vi "circ_ap && file_pgm.vi"() -> ()   [LabVIEW 2012, in "LightPipes.lvlib"]
uses:
  LightPipes.lvlib
panel:
  in  "n_grid":i32=256
  out "field out":T1
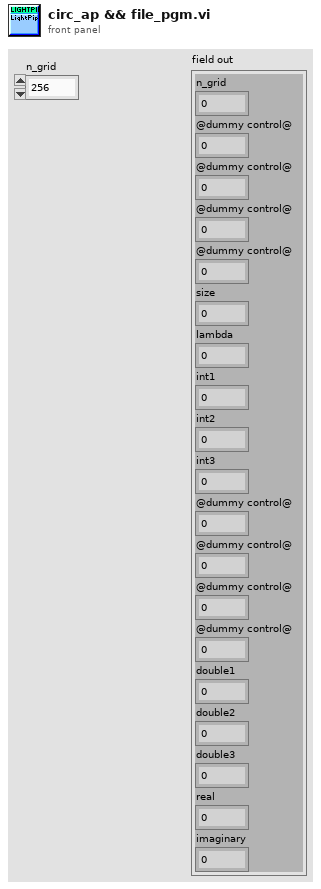
[diagram p1: front panel]
types:
  T1 = cluster{"n_grid":i32, "@dummy control@":i8, "@dummy control@":i8, "@dummy control@":i8, "@dummy control@":i8, "size":dbl, "lambda":dbl, "int1":i32, "int2":i32, "int3":i32, "@dummy control@":i8, "@dummy control@":i8, "@dummy control@":i8, "@dummy control@":i8, "double1":dbl, "double2":dbl, "double3":dbl, "real":u32, "imaginary":u32}
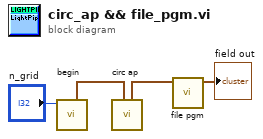
[diagram p0: block diagram]
diagram:
  n1 = call "begin.vi"("n_grid"="n_grid") -> ("field out"=w4:T1)  [unwired: 10 in]
  n2 = call "circ ap.vi"("field"=w4) -> ("field out"=w3:T1)  [unwired: 10 in]
  n3 = call "file pgm.vi"("field"=w3) -> ("field out"=→"field out":T1)  [unwired: 9 in, 1 out]
